vi "getRobotAxes.vi"(8 "error in":errorcluster) -> (0 "error out":errorcluster, 3 "Axes":dbl[](array[numeric]))   [LabVIEW 2013]
uses:
  ROS/Code/Console/Servers/ServerSubs/(nist) Arm Globals.vi
  CRCL Globals.vi
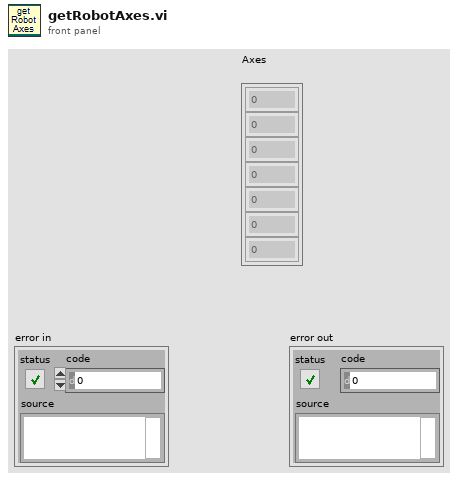
[diagram p1: front panel]
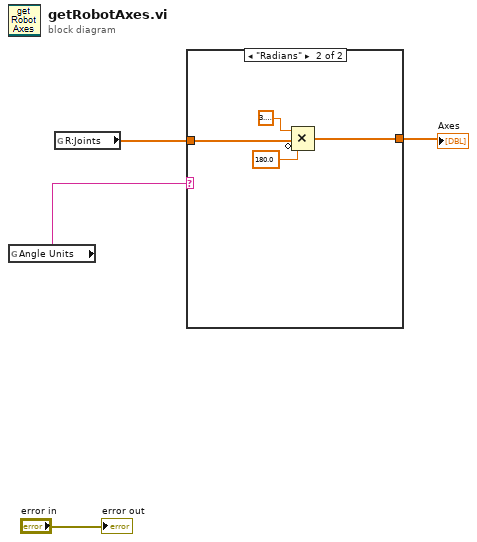
[diagram p0: block diagram]
diagram:
  n1 = global read "CRCL Globals.vi" "Angle Units"() -> (w3:string)
  n2 = global read "(nist) Arm Globals.vi" "R:Joints"() -> (w2:dbl[])
  n3 = case shown="\"Radians\"" w3 {
    tunnel: w2 -> [w5 w9]
    tunnel: [w5 w8] -> w1
    frame "Degrees", Default {
    }
    frame "Radians" {
      n4 = Compound Arithmetic op=MULTIPLY(3.141592653589793, w9, invert 180.0) -> (w8:dbl[])
    }
  }
  "Axes" <- w1
  "error out" <- "error in"
